vi "Dinner menu sub vi.vi"() -> ()   [LabVIEW 2019]
uses:
  Program Files (x86)/National Instruments/LabVIEW 2019/project/EN1Course-master (12)/EN1Course-master/_Subs/ThingWorx/_TW_Subs/TW_XControl.xctl
  Program Files (x86)/National Instruments/LabVIEW 2019/project/EN1Course-master (12)/EN1Course-master/_Subs/ThingWorx/_TW_Subs/Thingworx_Write_string.vi
panel:
  in  "MadDE2":string(xcontrol)="Day1:MadDE2"
  in  "MadDE1":string(xcontrol)="Day1:MadDE1"
  in  "MadCGS2":string(xcontrol)="Day1:MadCGS2"
  in  "MadCGS1":string(xcontrol)="Day1:MadCGS1"
  in  "MadDSS":string(xcontrol)="Day1:MadDSS"
  in  "MadDDES":string(xcontrol)="Day1:MadDDES"
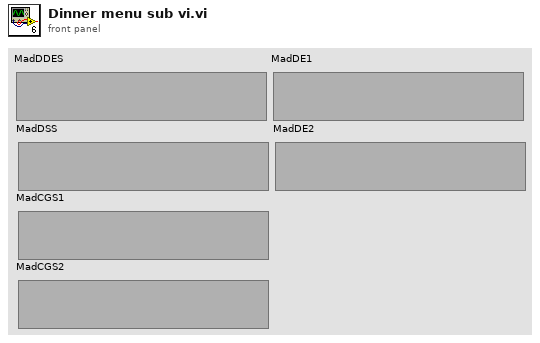
[diagram p1: front panel]
types:
  T1 = cluster{"menu-id":string, "data":cluster{"Dinner":cluster{"SPECIALTY SALADS":string[], "CHAR-GRILL STATIONS":string[], "FRESH BAKED DESSERTS":string[], "DINNER ENTREES":string[]}}}
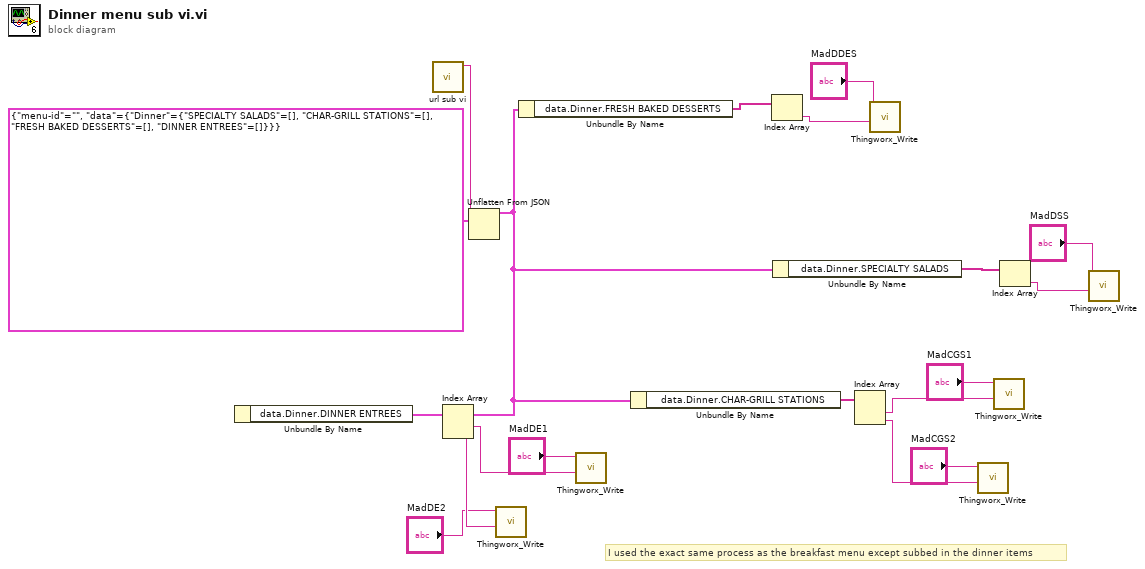
[diagram p0: block diagram]
diagram:
  # "I used the exact same process as the breakfast menu except subbed in the dinner items"
  n1 = call "url sub vi.vi"() -> ("body 2"=w19:string)  [unwired: 11 in]
  n2 = Unflatten From JSON(JSON string=w19, type and defaults=T1 {"menu-id"="", "data"={"Dinner"={"SPECIALTY SALADS"=[], "CHAR-GRILL STATIONS"=[], "FRESH BAKED DESSERTS"=[], "DINNER ENTREES"=[]}}}) -> (value=w17:T1)  [unwired: 5 in, 1 out]
  n3 = Unbundle By Name(w17) -> ("data.Dinner.DINNER ENTREES"=w15:string[])
  n4 = Index Array(array=w15) -> (element #1=w4:string, element #2=w2:string)  [unwired: 2 in]
  n5 = call-poly "Thingworx_Write.vi"("String"=w2, "Thingworx"="MadDE2") -> ()  [unwired: 10 in]
  n6 = Unbundle By Name(w17) -> ("data.Dinner.FRESH BAKED DESSERTS"=w13:string[])
  n7 = call-poly "Thingworx_Write.vi"("String"=w4, "Thingworx"="MadDE1") -> ()  [unwired: 10 in]
  n8 = Unbundle By Name(w17) -> ("data.Dinner.CHAR-GRILL STATIONS"=w16:string[])
  n9 = Index Array(array=w13) -> (element=w12:string)  [unwired: 1 in]
  n10 = Unbundle By Name(w17) -> ("data.Dinner.SPECIALTY SALADS"=w14:string[])
  n11 = Index Array(array=w16) -> (element #1=w8:string, element #2=w6:string)  [unwired: 2 in]
  n12 = call-poly "Thingworx_Write.vi"("String"=w12, "Thingworx"="MadDDES") -> ()  [unwired: 10 in]
  n13 = call-poly "Thingworx_Write.vi"("String"=w6, "Thingworx"="MadCGS2") -> ()  [unwired: 10 in]
  n14 = call-poly "Thingworx_Write.vi"("String"=w8, "Thingworx"="MadCGS1") -> ()  [unwired: 10 in]
  n15 = Index Array(array=w14) -> (element=w10:string)  [unwired: 1 in]
  n16 = call-poly "Thingworx_Write.vi"("String"=w10, "Thingworx"="MadDSS") -> ()  [unwired: 10 in]
